vi "Get Nested Enq.vi"(10 "Ident":string, 11 "Interactor in":refnum<class "Interactor.lvclass">) -> (1 "Enq":refnum<class "Message Enqueuer.lvclass">, 2 "Found?":bool, 3 "Interactor out":refnum<class "Interactor.lvclass">)   [LabVIEW 2024, in "Interactor.lvlib" / "Interactor.lvclass"]
uses:
  Interactor.lvclass
  <vilib>/ActorFramework/Message Enqueuer/Message Enqueuer.lvclass
  Interactor.lvclass/Interactor.ctl
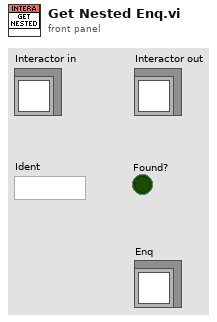
[diagram p1: front panel]
types:
  T1 = map{string, refnum<class "Message Enqueuer.lvclass">}
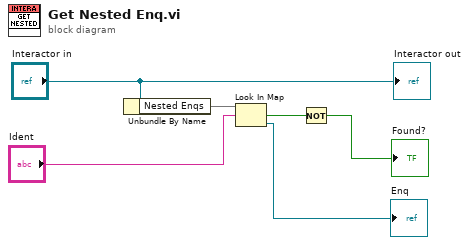
[diagram p0: block diagram]
diagram:
  n1 = Unbundle By Name("Interactor in") -> ("Nested Enqs"=w5:T1)
  n2 = Look In Map(map=w5, key="Ident") -> (key not found?=w3:bool, value=→"Enq":refnum<class "Message Enqueuer.lvclass">)  [unwired: 1 in]
  n3 = Not(x=w3) -> (.not. x?=→"Found?":bool)
  "Interactor out" <- "Interactor in"
